vi "concatinate 2 strings with linefeed.vi"(6 "String 2":string, 7 "String 1":string) -> (2 "Concatinated OUT":string)   [LabVIEW 2018]
doc: "THis VI concatinates 2 strings with a linefeed in between."
panel:
  # "[Title] - [DESCRIPTION]\n\nCopyright (C) 2004 Michael Aivaliotis michael@mmwis.com\n\nPlease visit http://www.OpenG.org to learn about the\nOpen Source LabVIEW software movement.\n\nThis library is free software; you can redistribute it and/or\nmodify it under the terms of the GNU Lesser General Public\nLicense as published by the Free Software Foundation; either\nversion 2.1 of the License, or (at your option) any later version.\nThis library is distributed in the hope that it will be useful,\nbut WITHOUT ANY WARRANTY; without even the implied warranty of\nMERCHANTABILITY or FITNESS FOR A PARTICULAR PURPOSE. See the GNU\nLesser General Public License for more details.\nYou should have received a copy of the GNU Lesser General Public\nLicense along with this library; if not, write to the Free Software\nFoundation, Inc., 59 Temple Place, Suite 330, Boston, MA 02111-1307 USA"
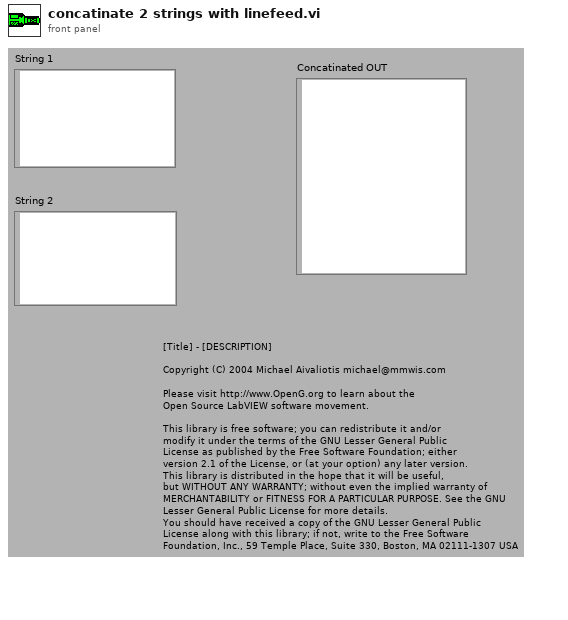
[diagram p1: front panel]
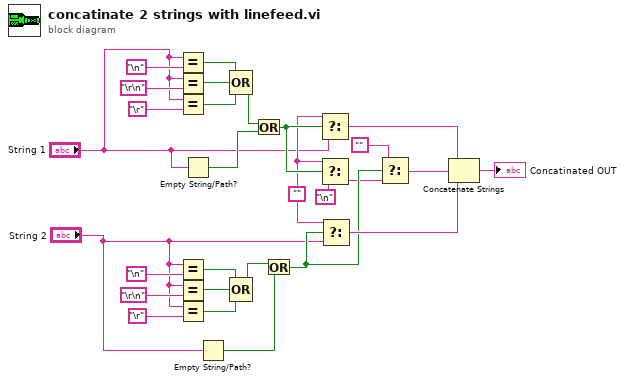
[diagram p0: block diagram]
diagram:
  w23 = ""
  n1 = Equal?(x="String 1", y="\n") -> (x = y?=w14:bool)
  n2 = Equal?(x="String 1", y="\r\n") -> (x = y?=w15:bool)
  n3 = Equal?(x="String 1", y="\r") -> (x = y?=w16:bool)
  n4 = Equal?(x="String 2", y="\n") -> (x = y?=w6:bool)
  n5 = Equal?(x="String 2", y="\r\n") -> (x = y?=w7:bool)
  n6 = Equal?(x="String 2", y="\r") -> (x = y?=w8:bool)
  n7 = Empty String/Path?(string/path="String 1") -> (empty?=w25:bool)
  n8 = Empty String/Path?(string/path="String 2") -> (empty?=w21:bool)
  n9 = Compound Arithmetic op=OR(w14, w15, w16) -> (w9:bool)
  n10 = Compound Arithmetic op=OR(w6, w7, w8) -> (w2:bool)
  n11 = Or(x=w9, y=w25) -> (x .or. y?=w24:bool)
  n12 = Or(x=w2, y=w21) -> (x .or. y?=w19:bool)
  n13 = Select(t=w23, s=w24, f="String 1") -> (s? t:f=w22:string)
  n14 = Select(t=w23, s=w24, f="\n") -> (s? t:f=w17:string)
  n15 = Select(t=w23, s=w19, f="String 2") -> (s? t:f=w27:string)
  n16 = Select(t="", s=w19, f=w17) -> (s? t:f=w20:string)
  n17 = Concatenate Strings(w22, w20, w27) -> (→"Concatinated OUT":string)
